vi "StateMachineSubVI.vi"(4 "releaseCube":bool, 6 "lift Cube":bool, 7 "opModeIsActive":bool, 9 "intakingCube":bool, 10 "haveCube":bool, 11 "done releasing cube":bool) -> ()   [LabVIEW 2017]
uses:
  Control 1.ctl
panel:
  in  "stop while loop":bool
  out "Current State":T1
  # "Note:  the boolean to stop a while loop is left there to stop the loop that would test the transitions of the states"
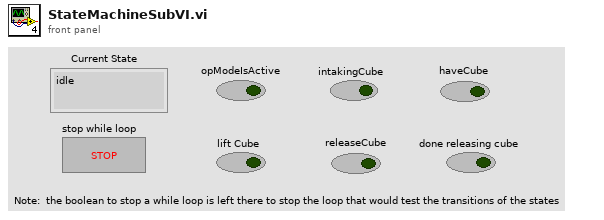
[diagram p1: front panel]
types:
  T1 = typedef "Control 1.ctl" = enum16{"idle", "takeInCube", "liftCube", "releaseCube", "haveCube", "doNothing"}
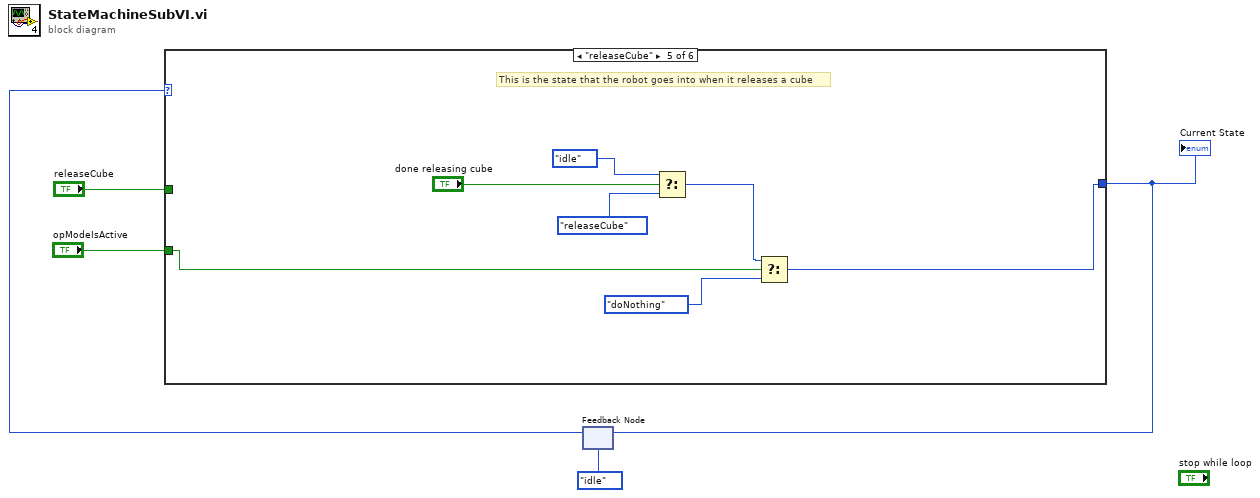
[diagram p0: block diagram]
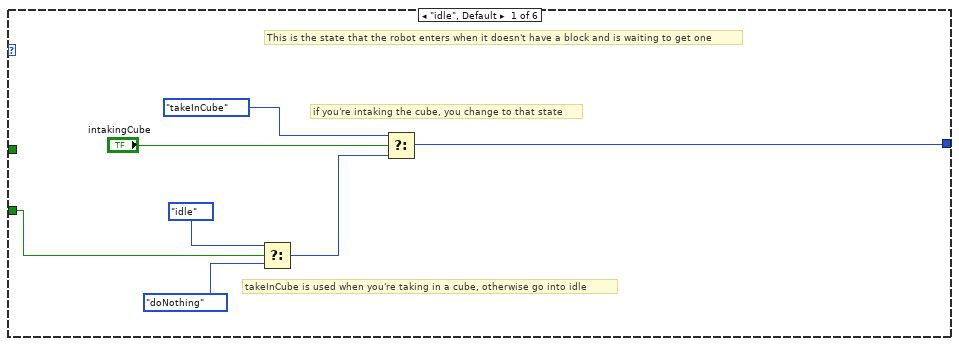
[diagram p2: hidden frame]
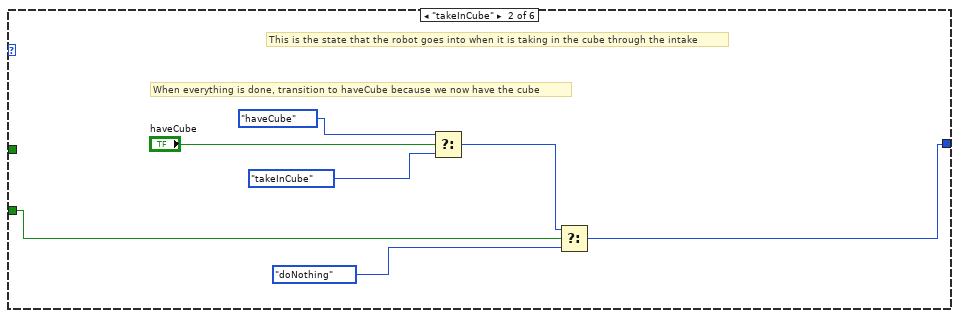
[diagram p3: hidden frame]
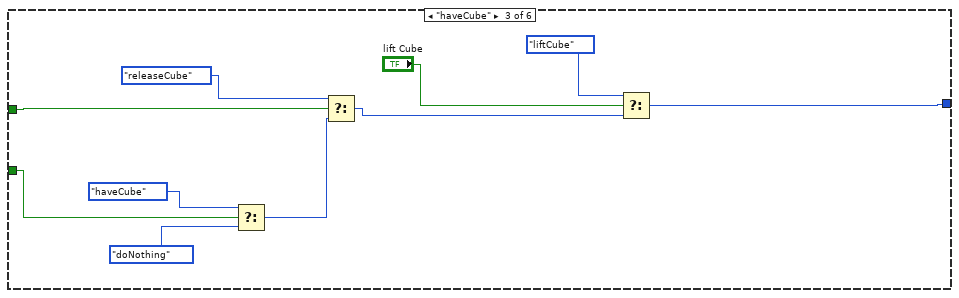
[diagram p4: hidden frame]
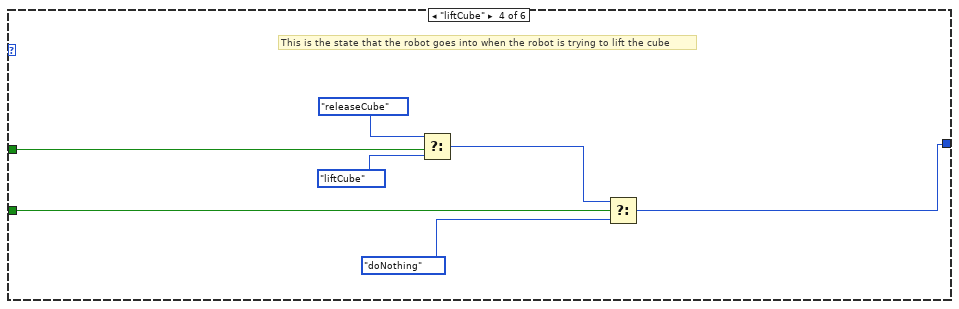
[diagram p5: hidden frame]
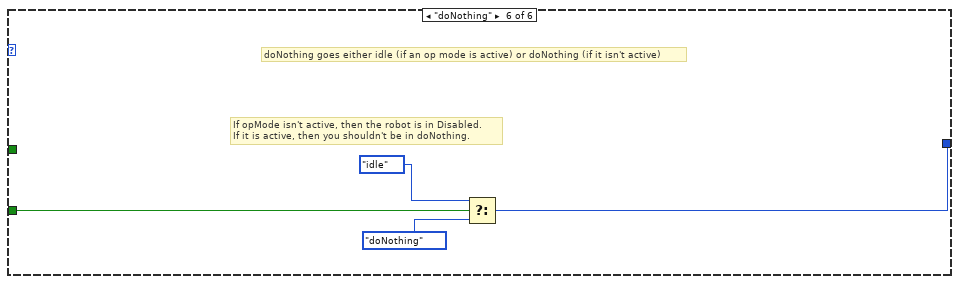
[diagram p6: hidden frame]
diagram:
  n1 = feedback #1(Control_1."idle") -> (w3:T1)
  n2 = case shown="\"releaseCube\"" w3 {
    tunnel: [w9 w14 w23 w32 w38 w45] -> w1
    tunnel: "releaseCube" -> [_ _ w25 w31 _ _]
    tunnel: "opModeIsActive" -> [w6 w13 w29 w30 w37 w44]
    frame "idle", Default {
      # "if you're intaking the cube, you change to that state"
      # "takeInCube is used when you're taking in a cube, otherwise go into idle"
      # "This is the state that the robot enters when it doesn't have a block and is waiting to get one"
      n3 = Select(t=Control_1."idle", s=w6, f=Control_1."doNothing") -> (s? t:f=w11:T1)
      n4 = Select(t=Control_1."takeInCube", s="intakingCube", f=w11) -> (s? t:f=w9:T1)
    }
    frame "takeInCube" {
      # "When everything is done, transition to haveCube because we now have the cube"
      # "This is the state that the robot goes into when it is taking in the cube through the intake"
      n5 = Select(t=Control_1."haveCube", s="haveCube", f=Control_1."takeInCube") -> (s? t:f=w16:T1)
      n6 = Select(t=w16, s=w13, f=Control_1."doNothing") -> (s? t:f=w14:T1)
    }
    frame "haveCube" {
      n7 = Select(t=Control_1."haveCube", s=w29, f=Control_1."doNothing") -> (s? t:f=w26:T1)
      n8 = Select(t=Control_1."releaseCube", s=w25, f=w26) -> (s? t:f=w22:T1)
      n9 = Select(t=Control_1."liftCube", s="lift Cube", f=w22) -> (s? t:f=w23:T1)
    }
    frame "liftCube" {
      # "This is the state that the robot goes into when the robot is trying to lift the cube"
      n10 = Select(t=Control_1."releaseCube", s=w31, f=Control_1."liftCube") -> (s? t:f=w34:T1)
      n11 = Select(t=w34, s=w30, f=Control_1."doNothing") -> (s? t:f=w32:T1)
    }
    frame "releaseCube" {
      # "This is the state that the robot goes into when it releases a cube"
      n12 = Select(t=Control_1."idle", s="done releasing cube", f=Control_1."releaseCube") -> (s? t:f=w40:T1)
      n13 = Select(t=w40, s=w37, f=Control_1."doNothing") -> (s? t:f=w38:T1)
    }
    frame "doNothing" {
      # "If opMode isn't active, then the robot is in Disabled.\nIf it is active, then you shouldn't be in doNothing."
      # "doNothing goes either idle (if an op mode is active) or doNothing (if it isn't active)"
      n14 = Select(t=Control_1."idle", s=w44, f=Control_1."doNothing") -> (s? t:f=w45:T1)
    }
  }
  "Current State" <- w1
  n15 = feedback-in #1(w1) -> ()
